vi "checkForErrorInjected.vi"(8 "error in (no error)":errorcluster, 11 "SMO.ErrorInjection in":refnum<class "SMO.ErrorInjection.lvclass">) -> (0 "error out":errorcluster, 3 "SMO.ErrorInjection dup":refnum<class "SMO.ErrorInjection.lvclass">)   [LabVIEW 2013, in "SMO.ErrorInjection.lvclass"]
uses:
  SMO.ErrorInjection.lvclass
  SMO.ErrorInjection.lvclass/SMO.ErrorInjection.ctl
  <vilib>/regexp/Match Regular Expression.xnode
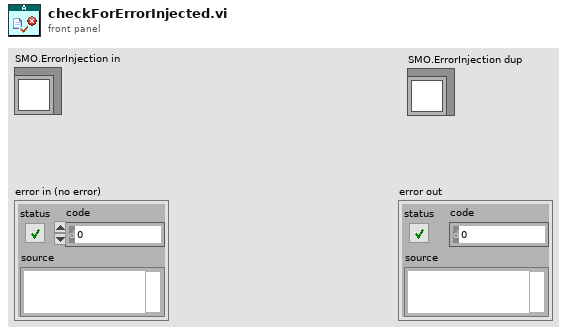
[diagram p1: front panel]
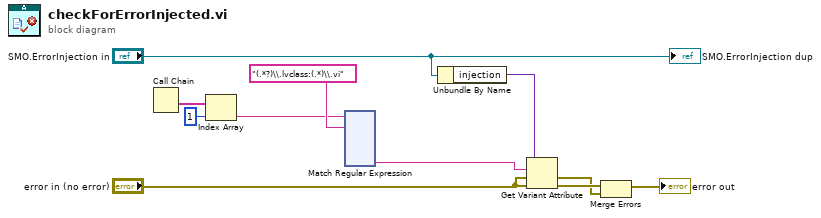
[diagram p0: block diagram]
diagram:
  n1 = Call Chain() -> (call chain=w5:string[])
  n2 = Index Array(array=w5, index=1) -> (element=w1:string)
  n3 = xnode "Match Regular Expression"("input string"=w1, "regular expression"="(.*?)\\.lvclass:(.*)\\.vi") -> ("submatch 2"=w2:string)  [unwired: 4 in, 6 out]
  n4 = Unbundle By Name("SMO.ErrorInjection in") -> ("injection"=w6:variant)
  n5 = Get Variant Attribute(Variant=w6, name=w2, default value (empty Variant)="error in (no error)", error in="error in (no error)") -> (value=w9:errorcluster, error out=w10:errorcluster)  [unwired: 2 out]
  n6 = Merge Errors(w10, w9) -> (→"error out":errorcluster)
  "SMO.ErrorInjection dup" <- "SMO.ErrorInjection in"
